vi "DAQ_Dig PWM Meas Close.vi"(0 "DAQmx Task In":refnum<k21>, 11 "error in":errorcluster) -> (15 "error out":errorcluster)   [LabVIEW 2021, in "DAQ_Digital PWM Measurement.lvlib"]
doc: "Aborts and clears the digital PWM measurement task"
uses:
  DAQ_Digital PWM Measurement.lvlib
panel:
  # "Inputs"
  # "Outputs"
  # "Overview:\nThis VI closes the digital PWM measurement DAQmx Task.\n\nHardware Requirement: TS-15050 DIO P0  \n\nSoftware Requirement: NI DAQmx 2022Q4 or later\n\nInstructions:\n1. Input the counter input measurement task through DAQmx Task In control.\n2. This VI aborts and clears the digital PWM measurement task."
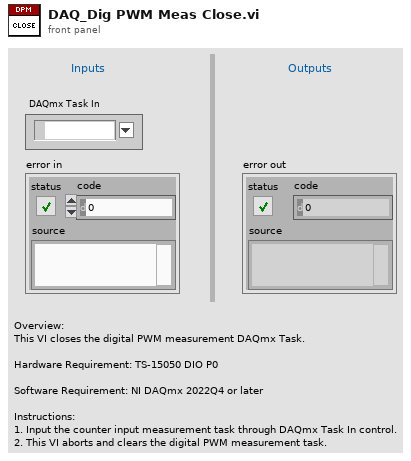
[diagram p1: front panel]
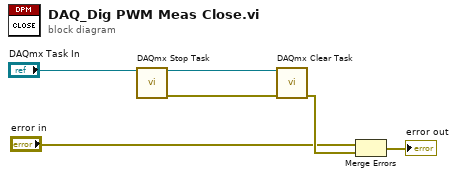
[diagram p0: block diagram]
diagram:
  n1 = call <vilib>:"DAQmx Stop Task.vi"("task/channels in"="DAQmx Task In") -> ("task out"=w5:refnum<k21>, "error out"=w4:errorcluster)  [unwired: 13 in]
  n2 = call <vilib>:"DAQmx Clear Task.vi"("task in"=w5, "error in"=w4) -> ("error out"=w2:errorcluster)  [unwired: 13 in]
  n3 = Merge Errors("error in", w2) -> (→"error out":errorcluster)
